vi "test.vi"() -> ()   [LabVIEW 2020]
panel:
  in  "stop":bool
  out "error out":errorcluster
  out "MEASure:VOLTage? CH2 Chart":dbl(graph)
  out "MEASure:VOLTage? CH1 Chart":dbl(graph)
  out "VISA resource name out":refnum<visa-resource-name>
  in  "error in":errorcluster
  in  "VISA resource name":refnum<visa-resource-name>
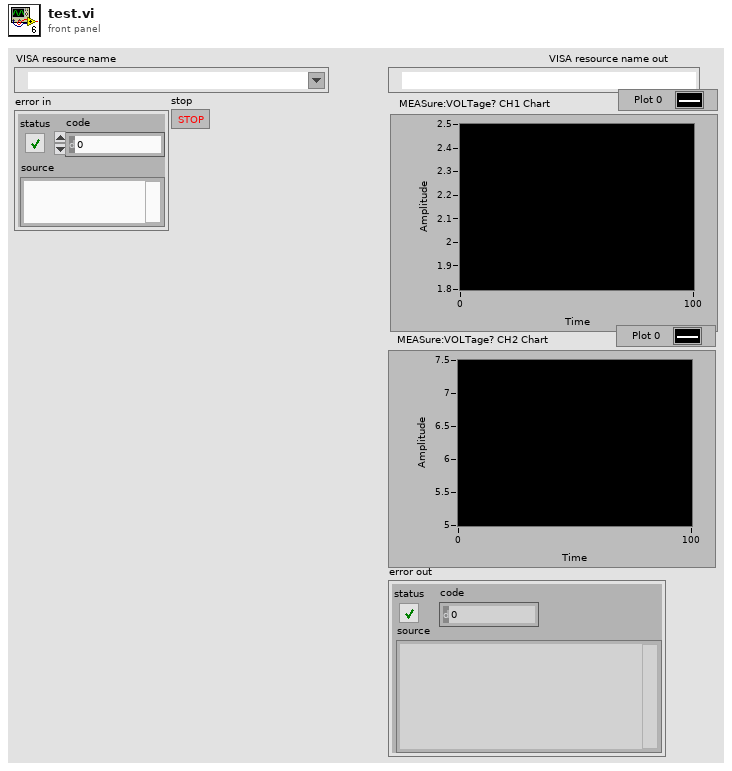
[diagram p1: front panel]
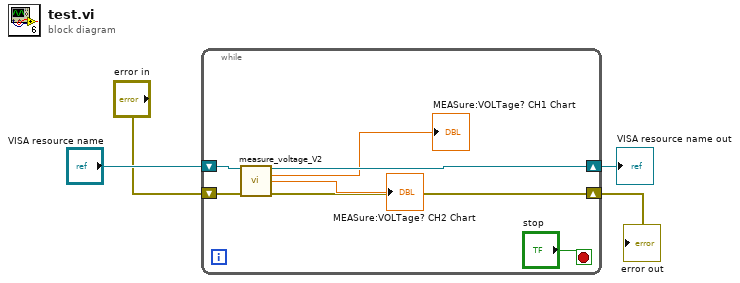
[diagram p0: block diagram]
diagram:
  n1 = while {
    shift-right: [w9] -> w2
    shift-left: "VISA resource name" -> [w11]
    shift-right: [w6] -> w1
    shift-left: "error in" -> [w10]
    stop <- "stop" stop-if-true
    n2 = call "measure_voltage_V2.vi"("VISA resource name"=w11, "error in"=w10) -> ("VISA resource name out"=w9:refnum<visa-resource-name>, "MEASure:VOLTage? CH1 Chart"=→"MEASure:VOLTage? CH1 Chart":dbl, "MEASure:VOLTage? CH2 Chart"=→"MEASure:VOLTage? CH2 Chart":dbl, "error out"=w6:errorcluster)  [unwired: 9 in, 1 out]
  }
  "VISA resource name out" <- w2
  "error out" <- w1
